vi "testARM.vi"() -> ()   [LabVIEW 2018]
panel:
  in  "fix to the line":bool
  in  "Enum":enum16{"forward", "backward", "left", "right"}(ring)
  in  "distance":dbl
  in  "speed":i32
  in  "Move robot":bool
  in  "push":bool
  in  "grip":bool
  in  "base":i32(slide) scale=-125.0..125.0
  in  "gripper":i32(slide)=128 step=1 scale=-90.0..90.0
  out "Encoder shoulder":i32
  out "Encoder elbow":i32
  in  "wrist angle":i32(slide) scale=-127.0..35.0
  out "elbow":bool
  out "shoulder":bool
  in  "elbow speed":i16
  in  "elbow angle":i32(slide) scale=-90.0..90.0
  in  "shoulder speed":i16
  in  "shoulder angle":i32(slide) scale=-30.0..40.0
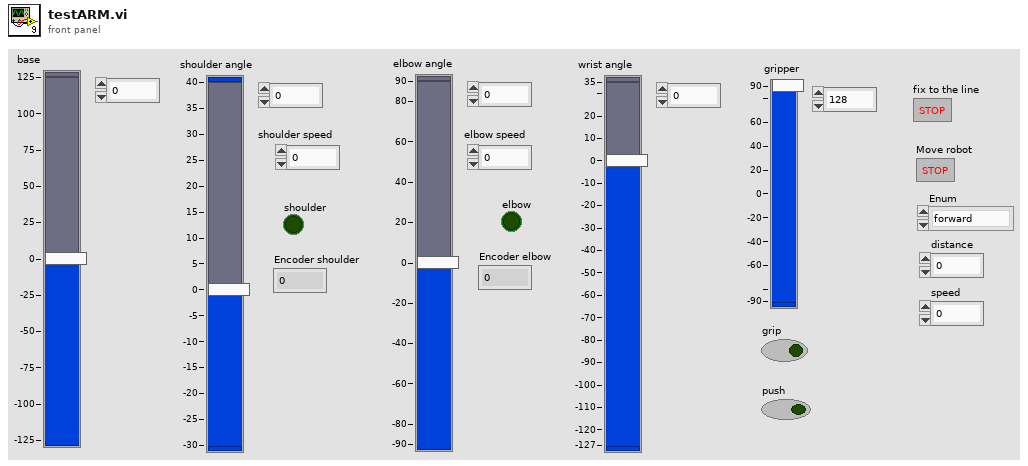
[diagram p1: front panel]
types:
  T1 = enum16{"shoulder", "elbow", "wrist", "base", "gripper"}
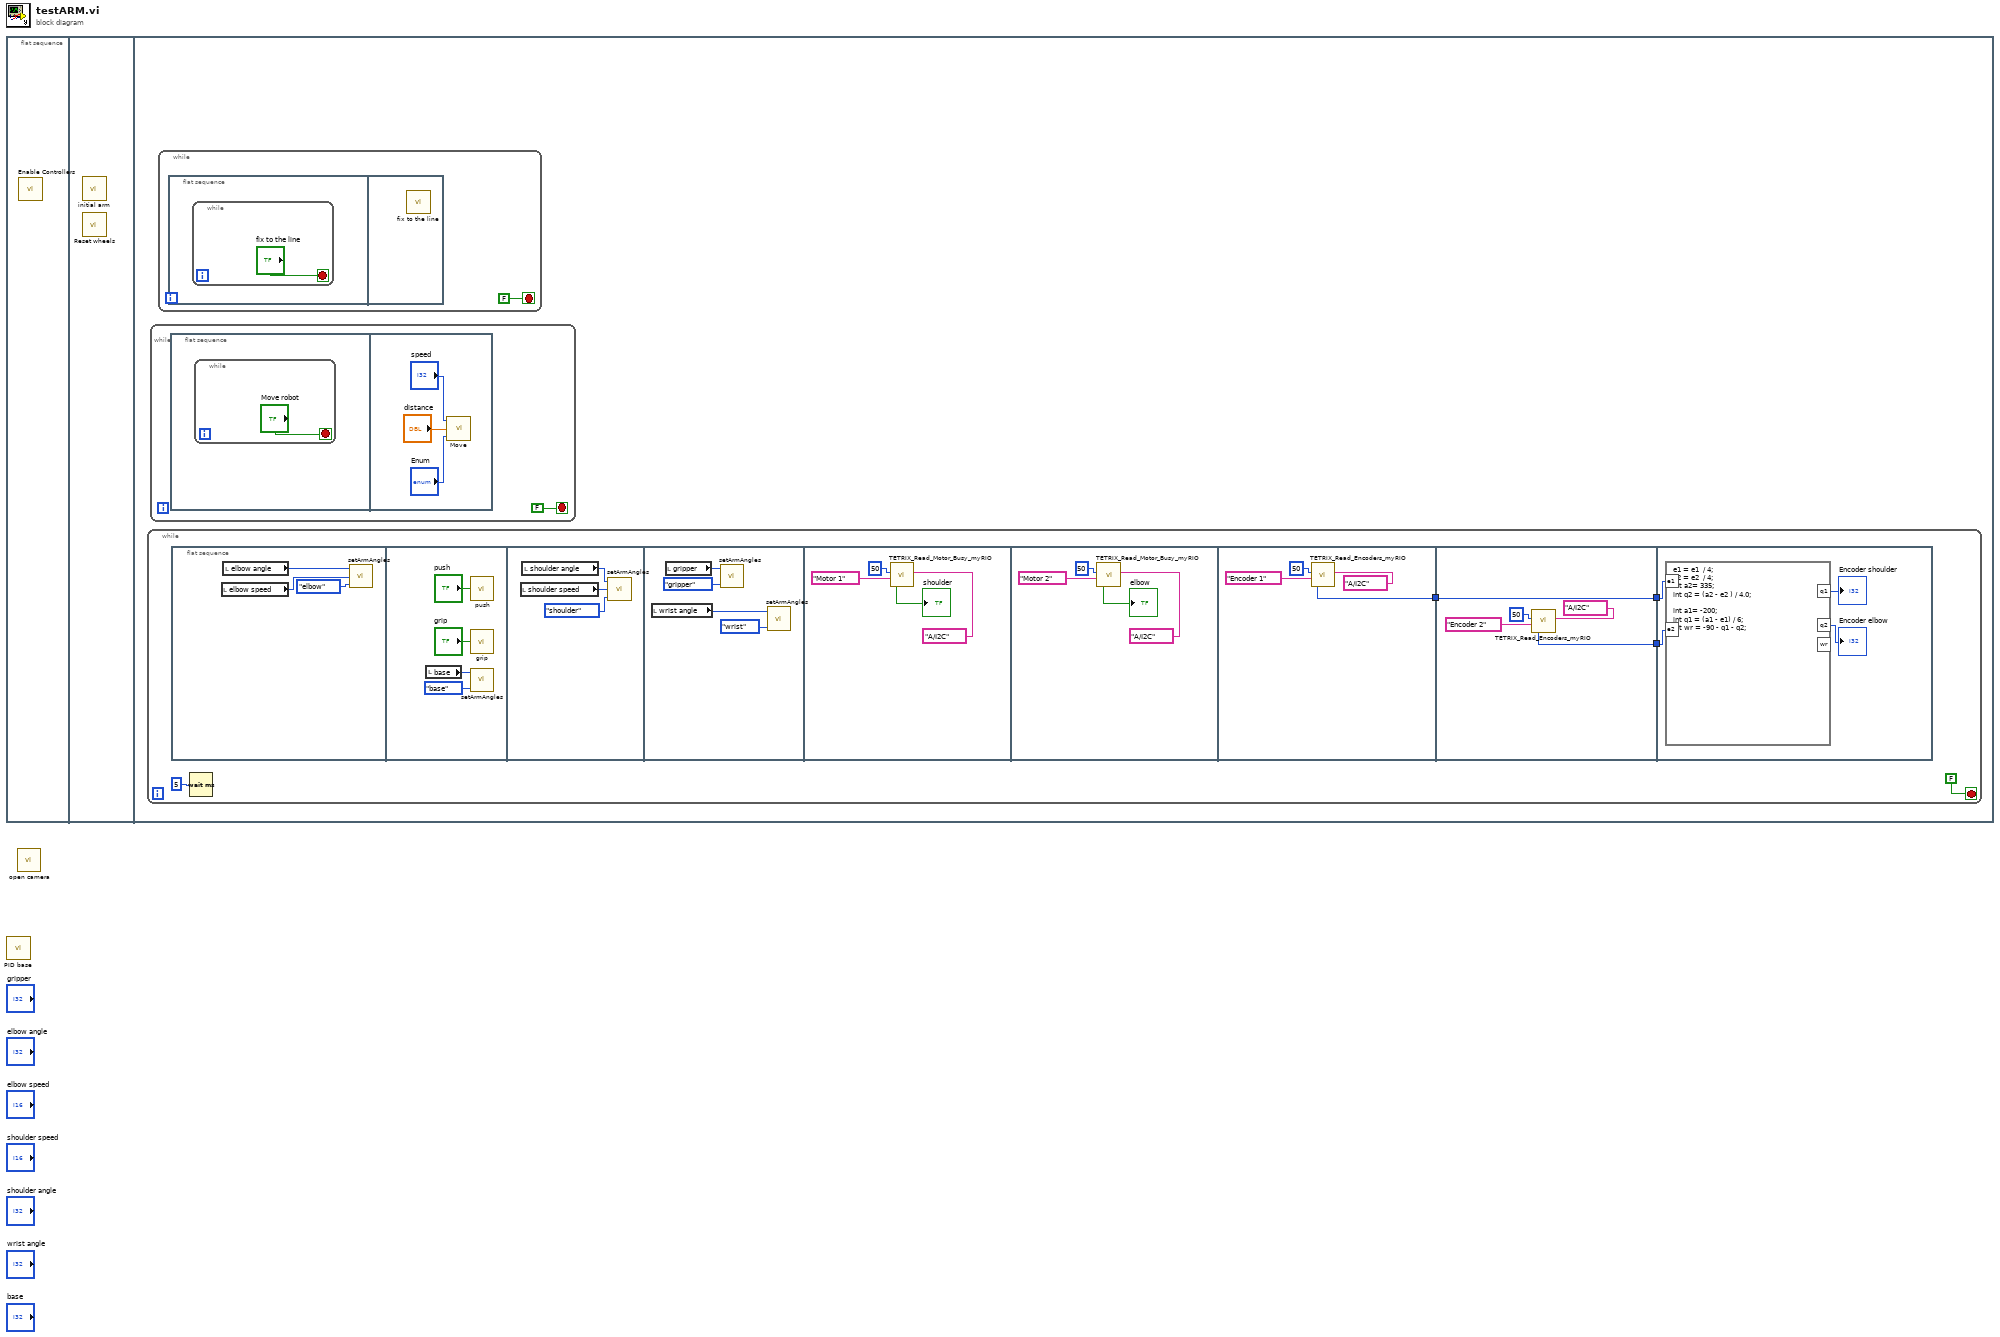
[diagram p0: block diagram]
diagram:
  n1 = flat-sequence {
    frame #0 {
      n2 = call "Enable Controllers.vi"() -> ()  [unwired: 12 in]
    }
    frame #1 {
      n3 = call "initial arm.vi"() -> ()  [unwired: 12 in]
      n4 = call "Reset wheels.vi"() -> ()  [unwired: 12 in]
    }
    frame #2 {
      n5 = while {
        stop <- FALSE stop-if-true
        n6 = flat-sequence {
          tunnel: [w35] -> w10
          tunnel: [w40] -> w11
          tunnel: w10 -> [w40]
          tunnel: [w39] -> w9
          tunnel: w11 -> [w45]
          tunnel: w9 -> [w44]
          frame #0 {
            n7 = local read "elbow speed"() -> (w14:i16)
            n8 = local read "elbow angle"() -> (w13:i32)
            n9 = call "setArmAngles.vi"("Enum"=enum16{"shoulder", "elbow"}."elbow", "speed"=w14, "angle"=w13) -> ()  [unwired: 1 in]
          }
          frame #1 {
            n10 = local read "base"() -> (w18:i32)
            n11 = call "push.vi"("push"="push") -> ()
            n12 = call "grip.vi"("grip"="grip") -> ()
            n13 = call "setArmAngles.vi"("Enum"=enum16{"shoulder", "elbow", "wrist", "base"}."base", "angle"=w18) -> ()  [unwired: 2 in]
          }
          frame #2 {
            n14 = local read "shoulder speed"() -> (w21:i16)
            n15 = local read "shoulder angle"() -> (w22:i32)
            n16 = call "setArmAngles.vi"("Enum"=enum16{"shoulder", "elbow"}."shoulder", "speed"=w21, "angle"=w22) -> ()  [unwired: 1 in]
          }
          frame #3 {
            n17 = local read "wrist angle"() -> (w25:i32)
            n18 = local read "gripper"() -> (w23:i32)
            n19 = call "setArmAngles.vi"("Enum"=T1."gripper", "angle"=w23) -> ()  [unwired: 2 in]
            n20 = call "setArmAngles.vi"("Enum"=enum16{"shoulder", "elbow", "wrist"}."wrist", "angle"=w25) -> ()  [unwired: 2 in]
          }
          frame #4 {
            n21 = call <vilib>:"TETRIX_Read_Motor_Busy_myRIO.vi"("myRIO MXP Port A/B"=tag "A/I2C", "Select Channel"="Motor 1", "Controller ID#  (I2C Address)"=u8 50) -> ("Motor Busy?"=→"shoulder":bool)  [unwired: 3 in, 1 out]
          }
          frame #5 {
            n22 = call <vilib>:"TETRIX_Read_Motor_Busy_myRIO.vi"("myRIO MXP Port A/B"=tag "A/I2C", "Select Channel"="Motor 2", "Controller ID#  (I2C Address)"=u8 50) -> ("Motor Busy?"=→"elbow":bool)  [unwired: 3 in, 1 out]
          }
          frame #6 {
            n23 = call <vilib>:"TETRIX_Read_Encoders_myRIO.vi"("myRIO MXP Port A/B"=tag "A/I2C", "Select Encoder"="Encoder 1", "Controller ID#  (I2C Address)"=u8 50) -> ("Encoder Output"=w35:i32)  [unwired: 3 in, 1 out]
          }
          frame #7 {
            n24 = call <vilib>:"TETRIX_Read_Encoders_myRIO.vi"("myRIO MXP Port A/B"=tag "A/I2C", "Select Encoder"="Encoder 2", "Controller ID#  (I2C Address)"=u8 50) -> ("Encoder Output"=w39:i32)  [unwired: 3 in, 1 out]
          }
          frame #8 {
            n25 = formula code="e1 = e1  / 4;\ne2 = e2  / 4;\nint a2= 335;\nint q2 = (a2 - e2 ) / 4.0;\n\nint a1= -200;\nint q1 = (a1 - e1) / 6;\nint wr = -90 - q1 - q2;"("e1"=w45, "e2"=w44) -> ("q1"=→"Encoder shoulder":i32, "q2"=→"Encoder elbow":i32)  [unwired: 1 out]
          }
        }
        n26 = Wait (ms)(milliseconds to wait=u32 5) -> ()  [unwired: 1 out]
      }
      n27 = while {
        stop <- FALSE stop-if-true
        n28 = flat-sequence {
          frame #0 {
            n29 = while {
              stop <- "Move robot" stop-if-true
            }
          }
          frame #1 {
            n30 = call "Move.vi"("Enum"="Enum", "distance"="distance", "speed"="speed") -> ()  [unwired: 1 in]
          }
        }
      }
      n31 = while {
        stop <- FALSE stop-if-true
        n32 = flat-sequence {
          frame #0 {
            n33 = while {
              stop <- "fix to the line" stop-if-true
            }
          }
          frame #1 {
            n34 = call "fix to the line.vi"() -> ()  [unwired: 12 in]
          }
        }
      }
    }
  }
  n35 = call "PID base.vi"() -> ()  [unwired: 12 in]
  n36 = call "open camera.vi"() -> ()  [unwired: 12 in]
